vi "ToggleJoystick.vi"(0 "object in":refnum<class "Prior_Zmotor.lvclass">, 2 "Enable(T)/Disable(F)":bool, 5 "error in (no error)":errorcluster) -> (14 "object out":refnum<class "Prior_Zmotor.lvclass">, 19 "error out":errorcluster)   [LabVIEW 2021, in "Prior_Zmotor.lvclass"]
uses:
  Prior_Zmotor.lvclass
  Prior_Zmotor.lvclass/Prior_Zmotor.ctl
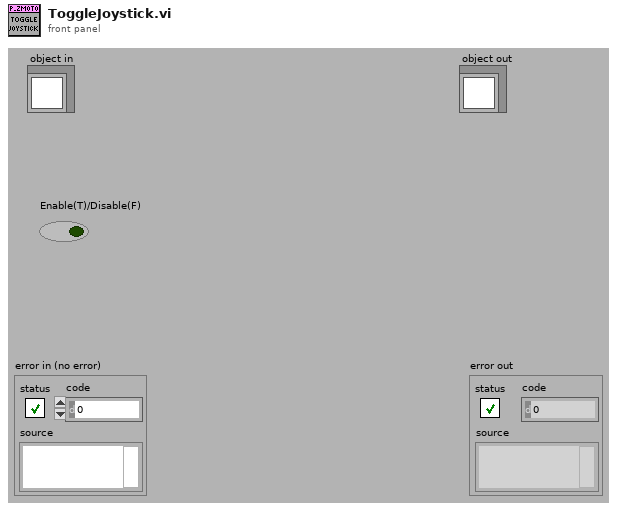
[diagram p1: front panel]
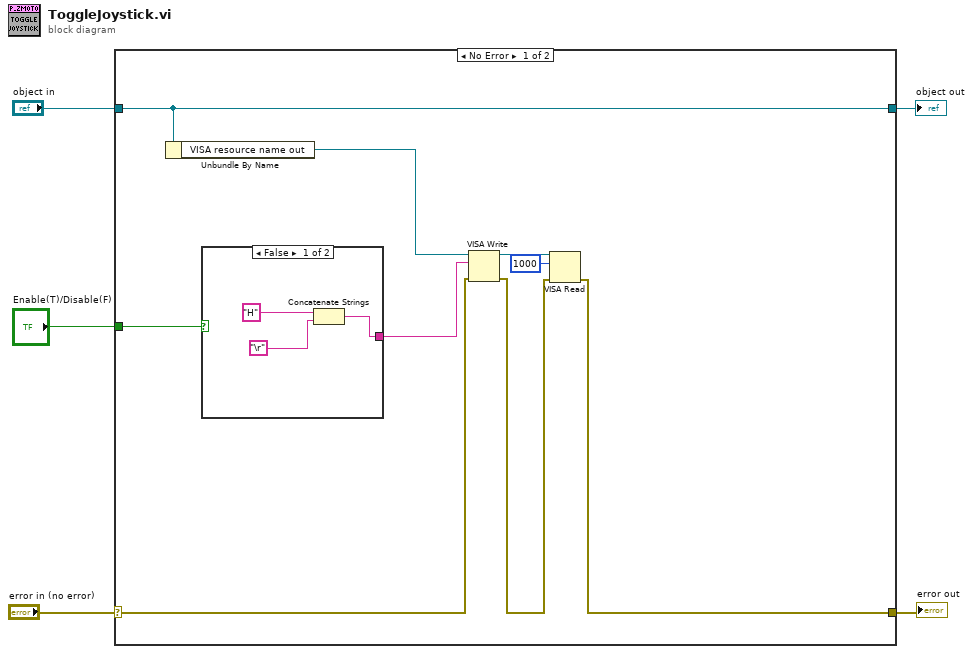
[diagram p0: block diagram]
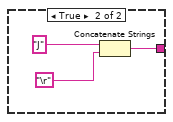
[diagram p2: hidden frame]
diagram:
  n1 = case shown="No Error" "error in (no error)" {
    selector: "error in (no error)" -> [w11 w22]
    tunnel: [w7 w22] -> w4
    tunnel: [w14 w21] -> w2
    tunnel: "object in" -> [w14 w21]
    tunnel: "Enable(T)/Disable(F)" -> [w10 _]
    frame No Error {
      n2 = Unbundle By Name(w14) -> ("VISA resource name out"=w13:refnum<visa-resource-name>)
      n3 = case shown="False" w10 {
        tunnel: [w15 w18] -> w12
        frame False {
          n4 = Concatenate Strings("H" ("write buffer"), "\r") -> (w15:string)
        }
        frame True {
          n5 = Concatenate Strings("J" ("write buffer"), "\r") -> (w18:string)
        }
      }
      n6 = VISA Write(VISA resource name=w13, write buffer=w12, error in (no error)=w11) -> (VISA resource name out=w9:refnum<visa-resource-name>, error out=w8:errorcluster)  [unwired: 1 out]
      n7 = VISA Read(VISA resource name=w9, byte count=u32 1000, error in (no error)=w8) -> (error out=w7:errorcluster)  [unwired: 3 out]
    }
    frame Error {
    }
  }
  "error out" <- w4
  "object out" <- w2
